vi "Connect.vi"(8 "error in (no error)":errorcluster, 9 "timeout in ms (10000)":i32=10000, 10 "General Settings":T2) -> (0 "error out":errorcluster, 3 "Local Queues":T1)   [LabVIEW 2020, in "Communication VIs.lvlib" / "Local.lvlib"]
uses:
  Local.lvlib
  Communication/IP_Communication/typedefs/General Settings.ctl
  Communication/IP_Communication/typedefs/Endpoint Tag.ctl
  Local Queues.ctl
  Communication/IP_Communication/IP_Communication.lvclass
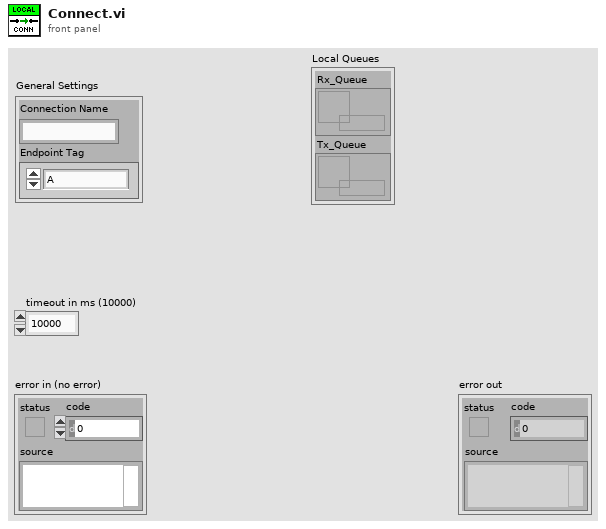
[diagram p1: front panel]
types:
  T1 = typedef "Communication VIs.lvlib/Local.lvlib/Local Queues.ctl" = cluster{"Rx_Queue":refnum<queue>, "Tx_Queue":refnum<queue>}
  T2 = typedef "Communication Classes.lvlib/IP_Communication.lvclass/General Settings.ctl" = cluster{"Connection Name":string, "Endpoint Tag":T3}
  T3 = typedef "Communication Classes.lvlib/IP_Communication.lvclass/Endpoint Tag.ctl" = enum8{"A", "B"}
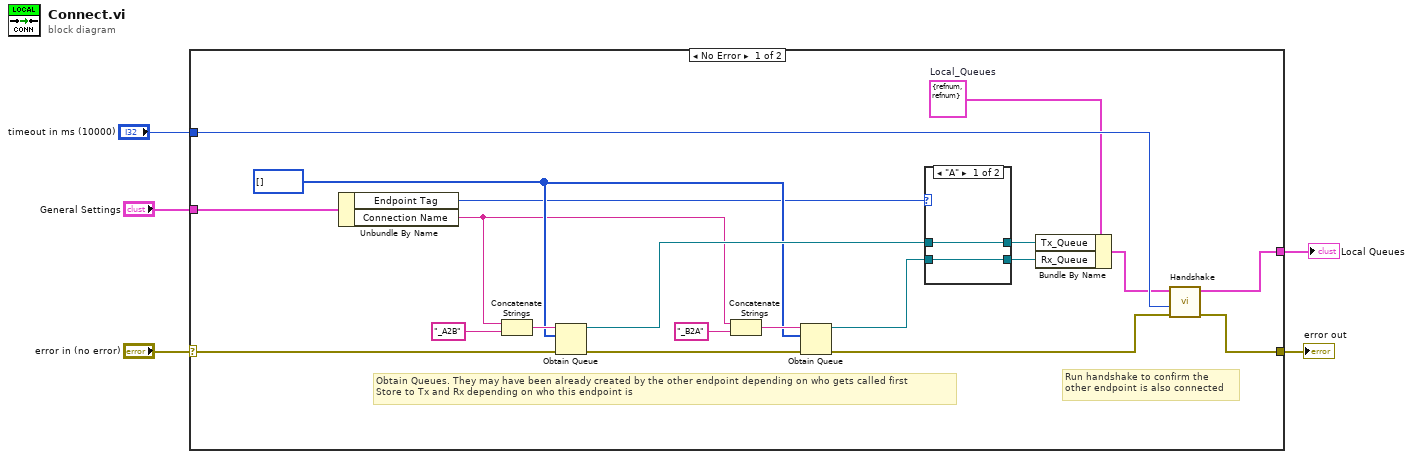
[diagram p0: block diagram]
diagram:
  n1 = case shown="No Error" "error in (no error)" {
    selector: "error in (no error)" -> [w17 w30]
    tunnel: "timeout in ms (10000)" -> [w11 _]
    tunnel: [w10 w30] -> w3
    tunnel: "General Settings" -> [w9 _]
    tunnel: [w6 _] -> w1
    frame No Error {
      w8 = T1 {"Rx_Queue"=refnum, "Tx_Queue"=refnum}  # Local_Queues
      w16 = u8[] []
      # "Run handshake to confirm the\nother endpoint is also connected"
      # "Obtain Queues. They may have been already created by the other endpoint depending on who gets called first\nStore to Tx and Rx depending on who this endpoint is"
      n2 = Unbundle By Name(w9) -> ("Endpoint Tag"=w13:T3, "Connection Name"=w14:string)
      n3 = Concatenate Strings(w14, "_A2B") -> (w24:string)
      n4 = Obtain Queue(name (unnamed)=w24, element data type=w16, error in (no error)=w17) -> (queue out=w22:refnum<queue>, error out=w15:errorcluster)  [unwired: 2 in, 1 out]
      n5 = Concatenate Strings(w14, "_B2A") -> (w23:string)
      n6 = Obtain Queue(name (unnamed)=w23, element data type=w16, error in (no error)=w15) -> (queue out=w21:refnum<queue>, error out=w12:errorcluster)  [unwired: 2 in, 1 out]
      n7 = case shown="\"A\"" w13 {
        tunnel: w22 -> [w27 w28]
        tunnel: w21 -> [w26 w29]
        tunnel: [w27 w29] -> w19
        tunnel: [w26 w28] -> w18
        frame "A" {
        }
        frame "B" {
        }
      }
      n8 = Bundle By Name(cluster=w8, "Tx_Queue"=w19, "Rx_Queue"=w18) -> (w7:T1)
      n9 = call "Handshake.vi"("error in (no error)"=w12, "timeout in ms (10000)"=w11, "Local Queues in"=w7) -> ("error out"=w10:errorcluster, "Local Queues out"=w6:T1)  [unwired: 7 in]
    }
    frame Error {
    }
  }
  "error out" <- w3
  "Local Queues" <- w1
